vi "SpliteString.vi"(2 "Split-Character":string, 3 "SourceStr":string) -> (0 "SubStr":string[](array[string]))   [LabVIEW 2018]
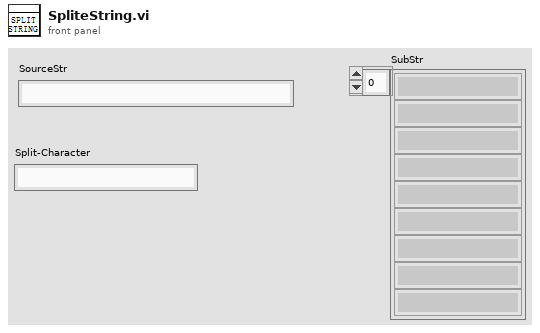
[diagram p1: front panel]
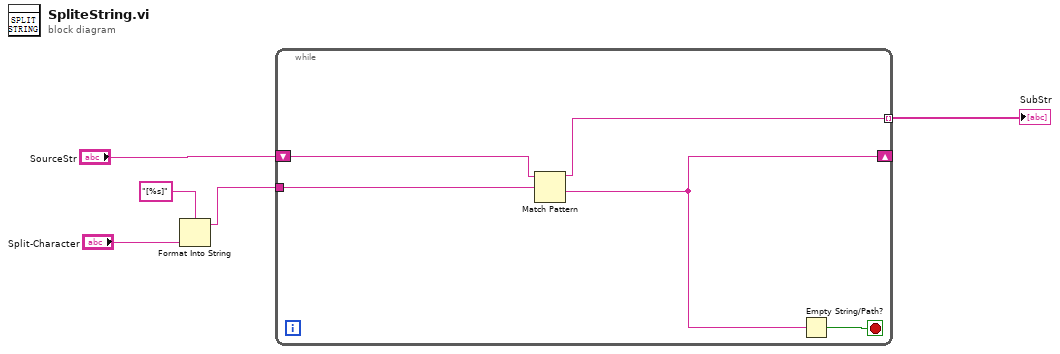
[diagram p0: block diagram]
diagram:
  n1 = Format Into String(format string="[%s]" ("格式字符串"), "Split-Character") -> (resulting string=w2:string)  [unwired: 2 in, 1 out]
  n2 = while {
    shift-right: [w8] -> _
    shift-left: "SourceStr" -> [w10]
    tunnel: w2 -> [w9]
    tunnel: [w6] -> w1 mode=indexing
    stop <- w7 stop-if-true
    n3 = Match Pattern(string=w10, regular expression=w9) -> (before substring=w6:string, after substring=w8:string)  [unwired: 1 in, 2 out]
    n4 = Empty String/Path?(string/path=w8) -> (empty?=w7:bool)
  }
  "SubStr" <- w1
